vi "Pot BBM.vi"(8 "error in":errorcluster, 11 "SyringeTool in":refnum<class "SyringeTool Class.lvclass">) -> (0 "error out":errorcluster, 3 "SyringeTool out":refnum<class "SyringeTool Class.lvclass">)   [LabVIEW 2011, in "SyringeTool Class.lvclass"]
uses:
  SyringeTool Class.lvclass
  WorkTable Class/WorkTable Class.lvclass
  Vec3d Class/Vec3d Class.lvclass
panel:
  in  "Slot":u32
  in  "Chuck":u32
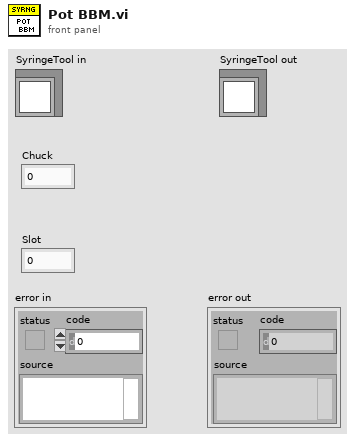
[diagram p1: front panel]
types:
  T1 = typedef "Worktable_BBM Slot.ctl" = cluster{"BBM Slot State":enum16{"Empty", "Unglued", "Stamped", "PartOnTop", "Weighted", "Unpotted", "Potted"}, "BBM Type":enum16{"BBM", "GlassSlide"}, "HDI Type":enum16{"HDI", "Polyimide"}, "Vacuum Channel":u8, "Location/Orientation BBM":T2, "Location/Orientation HDI":T2}
  T2 = typedef "Position_Orientation.ctl" = cluster{"Center":refnum<class "Vec3d Class.lvclass">, "Orientation":refnum<class "Orient3d Class.lvclass">}
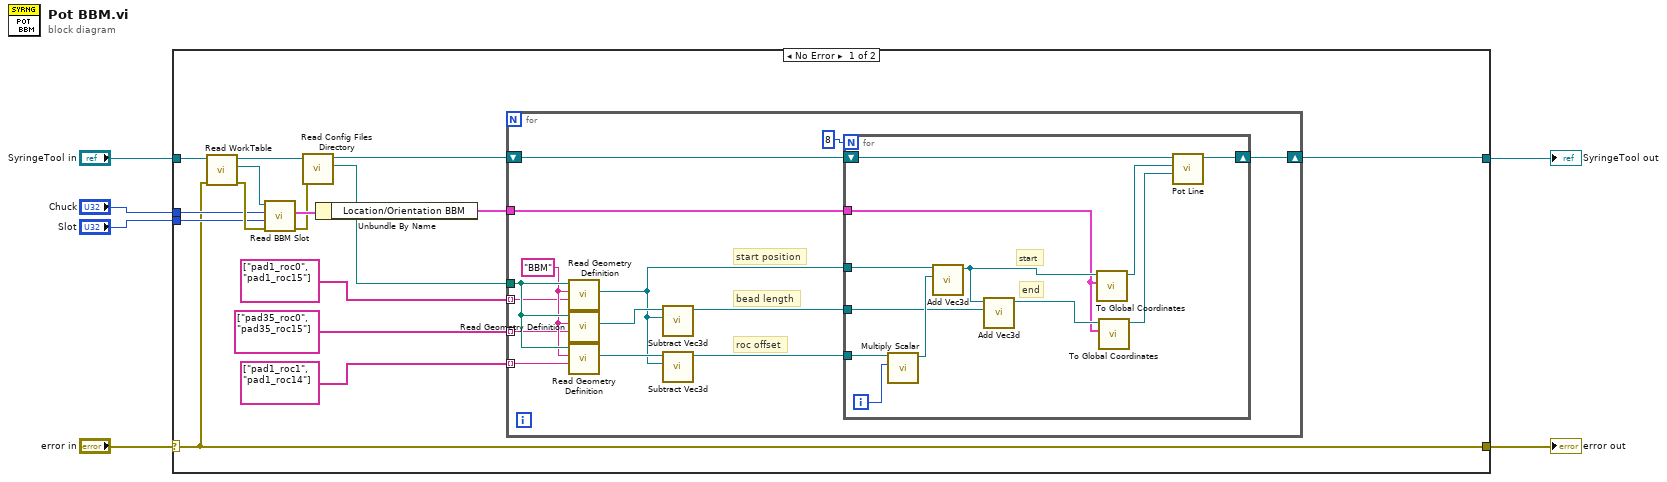
[diagram p0: block diagram]
diagram:
  n1 = case shown="No Error" "error in" {
    selector: "error in" -> [w7 w50]
    tunnel: [w7 w50] -> w5
    tunnel: [w11 w49] -> w3
    tunnel: "SyringeTool in" -> [w22 w49]
    tunnel: "Chuck" -> [w19 _]
    tunnel: "Slot" -> [w18 _]
    frame No Error {
      n2 = call-dynamic "Read WorkTable.vi"("error in"=w7, "Gantry Class in"=w22) -> ("error out"=w21:errorcluster, "WorkTable Class.lvclass"=w20:refnum<class "WorkTable Class.lvclass">, "Gantry Class out"=w16:refnum<class "SyringeTool Class.lvclass">)  [unwired: 7 in]
      n3 = call-dynamic "Read BBM Slot.vi"("error in (no error)"=w21, "Slot Number"=w18, "Chuck Number"=w19, "WorkTable Class in"=w20) -> ("error out"=w15:errorcluster, "BBM Slot"=w17:T1)  [unwired: 5 in, 1 out]
      n4 = call-dynamic "Read Config Files Directory.vi"("error in (no error)"=w15, "Gantry Class in"=w16) -> ("Config Files Directory"=w14:path, "Gantry Class out"=w12:refnum<class "SyringeTool Class.lvclass">)  [unwired: 7 in, 1 out]
      n5 = Unbundle By Name(w17) -> ("Location/Orientation BBM"=w13:T2)
      n6 = for {
        tunnel: w14 -> [w36]
        tunnel: string[] ["pad1_roc0", "pad1_roc15"] -> [w34] mode=indexing
        tunnel: string[] ["pad35_roc0", "pad35_roc15"] -> [w33] mode=indexing
        tunnel: string[] ["pad1_roc1", "pad1_roc14"] -> [w32] mode=indexing
        tunnel: w13 -> [w28]
        shift-right: [w23] -> w11
        shift-left: w12 -> [w24]
        w35 = "BBM" ("Part")
        # "roc offset"
        # "start position"
        # "bead length"
        n7 = call "Read Geometry Definition.vi"("Feature"=w34, "Part"=w35, "Config Location"=w36) -> ("Feature Coordinates"=w27:refnum<class "Vec3d Class.lvclass">)  [unwired: 7 in, 1 out]
        n8 = call "Read Geometry Definition.vi"("Feature"=w33, "Part"=w35, "Config Location"=w36) -> ("Feature Coordinates"=w31:refnum<class "Vec3d Class.lvclass">)  [unwired: 7 in, 1 out]
        n9 = call "Read Geometry Definition.vi"("Feature"=w32, "Part"=w35, "Config Location"=w36) -> ("Feature Coordinates"=w30:refnum<class "Vec3d Class.lvclass">)  [unwired: 7 in, 1 out]
        n10 = call "Subtract Vec3d.vi"("Vec3d in 2"=w27, "Vec3d in 1"=w31) -> ("Vec3d Class out"=w26:refnum<class "Vec3d Class.lvclass">)  [unwired: 8 in, 1 out]
        n11 = call "Subtract Vec3d.vi"("Vec3d in 2"=w27, "Vec3d in 1"=w30) -> ("Vec3d Class out"=w25:refnum<class "Vec3d Class.lvclass">)  [unwired: 8 in, 1 out]
        n12 = for {
          N: 8 -> [_]
          tunnel: w28 -> [w41]
          tunnel: w27 -> [w46]
          tunnel: w26 -> [w44]
          tunnel: w25 -> [w48]
          shift-right: [w37] -> w23
          shift-left: w24 -> [w38]
          i -> [w47]
          # "end"
          # "start"
          n13 = call-dynamic "Multiply Scalar.vi"("Scale"=w47, "Vec3d in"=w48) -> ("Vec3d out"=w45:refnum<class "Vec3d Class.lvclass">)  [unwired: 8 in, 1 out]
          n14 = call-dynamic "Add Vec3d.vi"(10:"Vec3d Class in"=w45, 11:"Vec3d Class in"=w46) -> ("Vec3d Class out"=w43:refnum<class "Vec3d Class.lvclass">)  [unwired: 8 in, 1 out]
          n15 = call-dynamic "Add Vec3d.vi"(10:"Vec3d Class in"=w44, 11:"Vec3d Class in"=w43) -> ("Vec3d Class out"=w42:refnum<class "Vec3d Class.lvclass">)  [unwired: 8 in, 1 out]
          n16 = call "To Global Coordinates.vi"("Center/Orientation"=w41, "Local Coordinates"=w43) -> ("Global Coordinates"=w40:refnum<class "Vec3d Class.lvclass">)  [unwired: 8 in, 1 out]
          n17 = call "To Global Coordinates.vi"("Center/Orientation"=w41, "Local Coordinates"=w42) -> ("Global Coordinates"=w39:refnum<class "Vec3d Class.lvclass">)  [unwired: 8 in, 1 out]
          n18 = call-dynamic "Pot Line.vi"("End Position"=w39, "Start Position"=w40, "SyringeTool in"=w38) -> ("SyringeTool out"=w37:refnum<class "SyringeTool Class.lvclass">)  [unwired: 7 in, 1 out]
        }
      }
    }
    frame Error {
    }
  }
  "error out" <- w5
  "SyringeTool out" <- w3
